vi "Get SOC OCV Curve.vi"(0 "reference in":refnum<class "Battery.lvclass">, 5 "Error In":errorcluster) -> (14 "reference out":refnum<class "Battery.lvclass">, 16 "SOC OCV Curve":dbl[][](array[numeric]), 19 "Error Out":errorcluster)   [LabVIEW 2023, in "Battery.lvclass"]
uses:
  Battery.lvclass
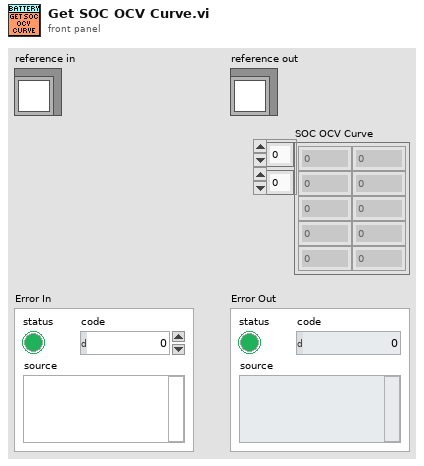
[diagram p1: front panel]
types:
  T1 = typedef "Battery.lvclass/ObjectAttributes.ctl" = cluster{"Python module":path, "Python Session":refnum<k35>, "PybammWrapper":refnum<k38>, "model loaded":bool, "simulation loaded":bool, "simulation enabled":bool, "SOC OCV Curve":dbl[][], "Open Circuit Voltage (V)":dbl, "State of Charge (%)":dbl}
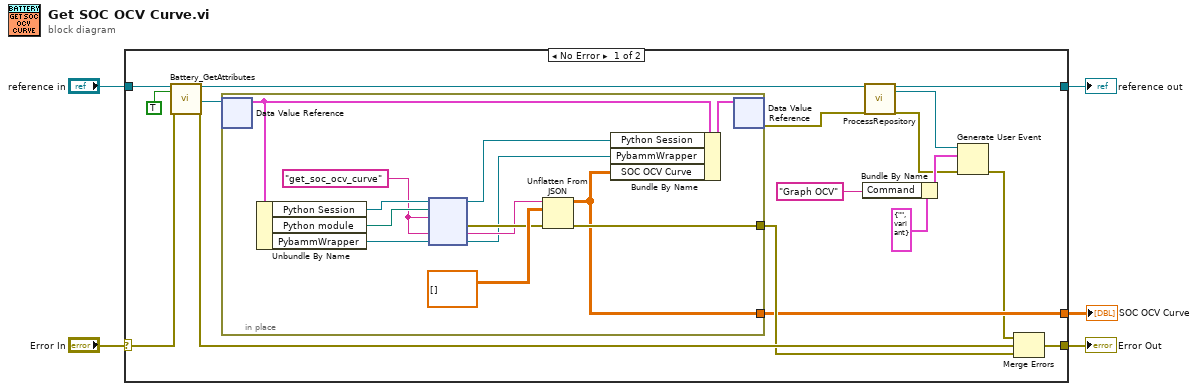
[diagram p0: block diagram]
diagram:
  n1 = case shown="No Error" "Error In" {
    selector: "Error In" -> [w22 w37]
    tunnel: [w21 w37] -> w4
    tunnel: [w8 w36] -> w2
    tunnel: "reference in" -> [w15 w36]
    tunnel: [w16 _] -> w1
    frame No Error {
      n2 = call "Battery_GetAttributes.vi"("reference in"=w15, "OnlyGetDvrReference(False)"=TRUE, "Error In"=w22) -> ("reference out"=w9:refnum<class "Battery.lvclass">, "DataRef"=w20:refnum<data-value>, "Error Out"=w18:errorcluster)  [unwired: 13 in, 1 out]
      n3 = in-place {
        in-place-border: [w26] -> w17
        in-place-border: [w25] -> w16
        w29 = "get_soc_ocv_curve" ("function name")
        n4 = in-place-dvr #1(w20) -> (w34:T1)  [unwired: 1 out]
        n5 = Unbundle By Name(w34) -> ("Python Session"=w32:refnum<k35>, "Python module"=w31:path, "PybammWrapper"=w33:refnum<k38>)
        n6 = node(w32, w31, w29, w29, w33) -> (w23:refnum<k35>, w28:errorcluster, w27:string, w24:refnum<k38>)  [unwired: 1 in, 2 out]
        n7 = Unflatten From JSON(JSON string=w27, type and defaults=dbl[][] [], error in (no error)=w28) -> (value=w25:dbl[][], error out=w26:errorcluster)  [unwired: 4 in]
        n8 = Bundle By Name(cluster=w34, "Python Session"=w23, "PybammWrapper"=w24, "SOC OCV Curve"=w25) -> (w35:T1)
        n9 = in-place-dvr #1(w35) -> (w6:errorcluster)  [unwired: 1 out]
      }
      n10 = Bundle By Name(cluster=cluster{"Command":string, "Data":variant} {"Command"="", "Data"=variant} ("MessageToProcess"), "Command"="Graph OCV") -> (w14:cluster{"Command":string, "Data":variant})
      n11 = call "ProcessRepository.vi"("reference in"=w9, "Error In"=w6) -> ("reference out"=w8:refnum<class "Battery.lvclass">, "EventsToProcess"=w12:refnum<user-event>, "Error Out"=w13:errorcluster)  [unwired: 10 in, 5 out]
      n12 = Generate User Event(user event=w12, event data cluster=w14, error in=w13) -> (error out=w7:errorcluster)  [unwired: 1 in, 1 out]
      n13 = Merge Errors(w7, w18, w17) -> (w21:errorcluster)
    }
    frame Error {
    }
  }
  "Error Out" <- w4
  "reference out" <- w2
  "SOC OCV Curve" <- w1
